vi "StepperGoHome.vi"(7 "PulseCounterChanel":T1=enum."CH4", 8 "Error In":errorcluster) -> (0 "Error Out":errorcluster, 3 "PulseCount":i32)   [LabVIEW 2019]
uses:
  WSCbot_V3_Toolkit.lvlibp/WSCBOTV3_Toolkit/IO/LowLevel/PulseCounter.ctl
  <vilib>/Platform/TimedLoop/XDataNode/timing_clust.ctl
  <vilib>/Platform/TimedLoop/XDataNode/nitl_modes.ctl
  <vilib>/Platform/TimedLoop/XDataNode/wakeup.ctl
  WSCbot_V3_Toolkit.lvlibp/WSCBOTV3_Toolkit/IO/LowLevel/IO_Chanel_DIO.ctl
  <vilib>/platform/TimedLoop/XDataNode/XDataNode.xnode
  <vilib>/Platform/TimedLoop/XDataNode/XDNodeRunTimeDep.lvlib
  WSCbot_V3_Toolkit.lvlibp
panel:
  in  "Stop Button":bool
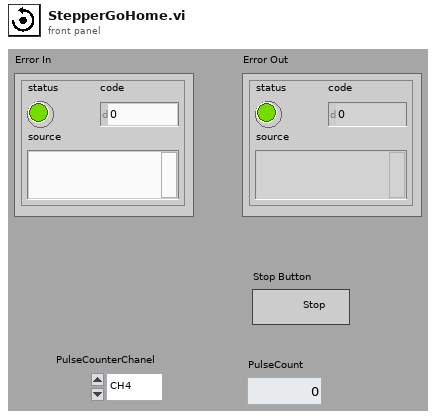
[diagram p1: front panel]
types:
  T1 = typedef "WSCbot_V3_Toolkit.lvlibp/PulseCounter.ctl" = enum16{"CH1", "CH2", "CH3", "CH4", "CH5"}
  T2 = typedef "XDNodeRunTimeDep.lvlib/timing_clust.ctl" = cluster{"Expected End [f-1]":u64, "Actual End [f-1]":u64, "Finished Late? [f-1]":bool, "Expected End [i-1]":u64, "Actual End [i-1]":u64, "Finished Late? [i-1]":bool, "Expected Start [i]":u64, "Actual Start [i]":u64, "Expected Start [f]":u64, "Actual Start [f]":u64, "Source Name":string, "Structure Name":string, "Period":i64, "Deadline":i64, "Offset":i64, "Start":i64, "Priority":i32, "Timeout":i32, "Mode":T3, "Wakeup Reason":T4, "Error":errorcluster, "Source Type":string, "Secondary Source Type":string, "Global End Time":u64, "Global Start Time":u64, "Frame Duration":u64, "Iteration Duration":u64, "Assigned CPU":i32, "I/O Scan Engine Mode":u32}
  T3 = typedef "XDNodeRunTimeDep.lvlib/nitl_modes.ctl" = enum32{"No Change", "Process missed periods, maintain original phase", "Discard missed periods, maintain original phase", "Process missed periods, ignore original phase", "Discard missed periods, ignore original phase"}
  T4 = typedef "XDNodeRunTimeDep.lvlib/wakeup.ctl" = enum32{"Normal", "Aborted", "Asynchronous wakeup", "Timing source error", "Timed loop error", "Timeout"}
  T5 = typedef "WSCbot_V3_Toolkit.lvlibp/IO_Chanel_DIO.ctl" = enum16{"A/DIO9", "A/DIO10", "C/DIO0", "C/DIO1", "C/DIO2", "C/DIO3", "C/DIO4", "C/DIO5", "C/DIO6"}
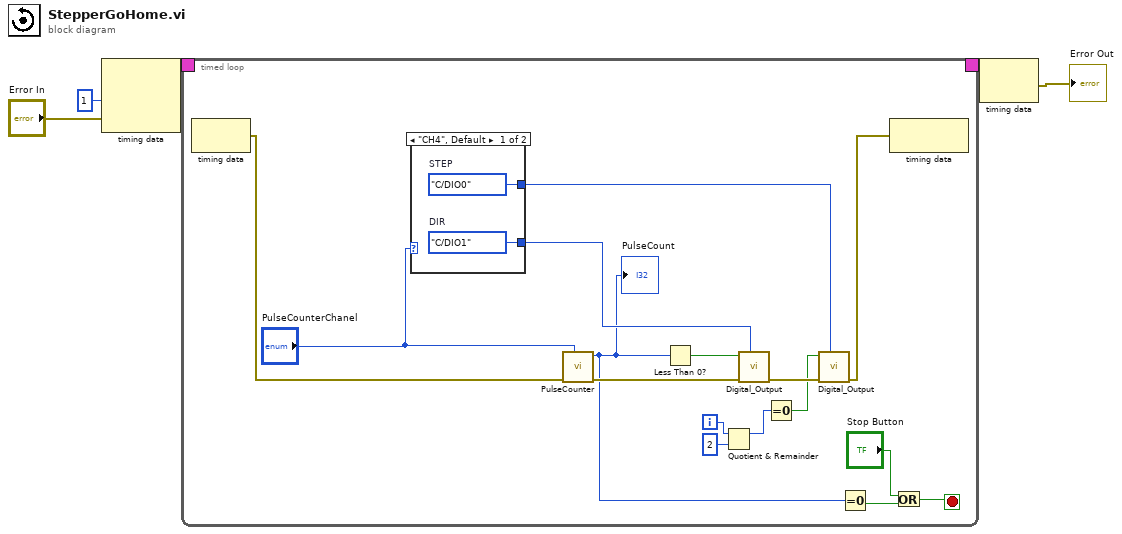
[diagram p0: block diagram]
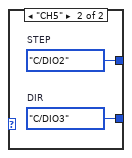
[diagram p2: hidden frame]
diagram:
  n1 = node-c288(i64 1 ("Period"), "Error In") -> (w5:T2)  [unwired: 1 in]
  n2 = timed-loop {
    timing: w5 -> [_]
    timing-out: [_] -> w4
    i -> [w20]
    stop <- w9 stop-if-true
    n3 = node-c288() -> (w6:errorcluster)  [unwired: 1 in]
    n4 = case shown="\"CH4\", Default" "PulseCounterChanel" {
      tunnel: [w23 w25] -> w16
      tunnel: [w22 w24] -> w15
      frame "CH4", Default {
        w23 = IO_Chanel_DIO."C/DIO1"  # DIR
        w22 = IO_Chanel_DIO."C/DIO0"  # STEP
      }
      frame "CH5" {
        w25 = IO_Chanel_DIO."C/DIO3"  # DIR
        w24 = IO_Chanel_DIO."C/DIO2"  # STEP
      }
    }
    n5 = call "PulseCounter.vi"("PulseCounterChanel"="PulseCounterChanel", "error in"=w6) -> ("error out"=w13:errorcluster, "PulseCount"=w7:i32)  [unwired: 8 in]
    "PulseCount" <- w7
    n6 = Less Than 0?(x=w7) -> (x < 0?=w11:bool)
    n7 = Quotient & Remainder(x=w20, y=2) -> (x-y*floor(x/y)=w18:i32)  [unwired: 1 out]
    n8 = call "Digital_Output.vi"("IO_Chanel"=w16, "error in"=w13, "False/True"=w11) -> ("error out"=w21:errorcluster)  [unwired: 8 in]
    n9 = Equal To 0?(x=w18) -> (x = 0?=w14:bool)
    n10 = call "Digital_Output.vi"("IO_Chanel"=w15, "error in"=w21, "False/True"=w14) -> ("error out"=w12:errorcluster)  [unwired: 8 in]
    n11 = Equal To 0?(x=w7) -> (x = 0?=w8:bool)
    n12 = node-c288(w12) -> ()  [unwired: 1 out]
    n13 = Or(x="Stop Button", y=w8) -> (x .or. y?=w9:bool)
  }
  n14 = node-c288(w4) -> (→"Error Out":errorcluster)
